vi "Add VI.vi"(8 "error in (no error)":errorcluster, 10 "Path":path, 11 "Project in":refnum<class "Project.lvclass">) -> (0 "error out":errorcluster, 3 "Project out":refnum<class "Project.lvclass">)   [LabVIEW 2015, in "Project.lvclass"]
uses:
  Project.lvclass
  Project.lvclass/Project.ctl
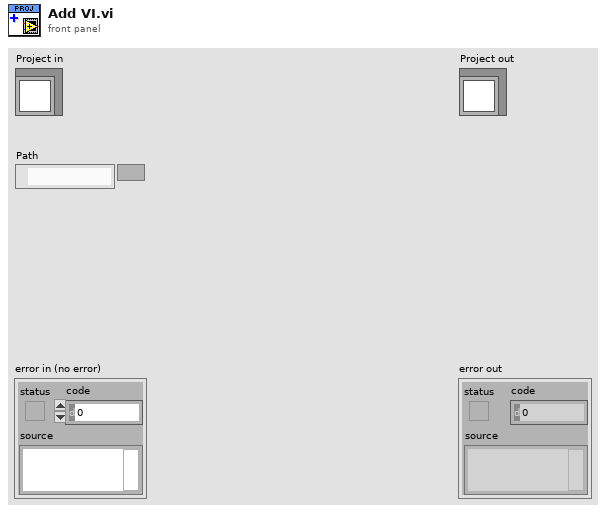
[diagram p1: front panel]
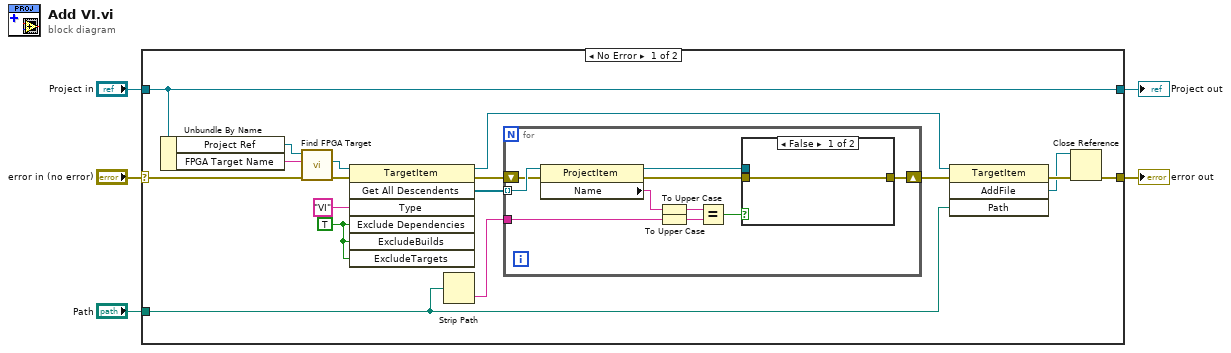
[diagram p0: block diagram]
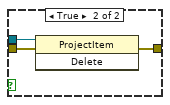
[diagram p2: hidden frame]
diagram:
  n1 = case shown="No Error" "error in (no error)" {
    selector: "error in (no error)" -> [w19 w38]
    tunnel: [w17 w38] -> w4
    tunnel: [w22 w37] -> w2
    tunnel: "Project in" -> [w22 w37]
    tunnel: "Path" -> [w8 _]
    frame No Error {
      w13 = TRUE ("ExcludeDependencies")
      n2 = Unbundle By Name(w22) -> ("Project Ref"=w21:refnum<vi>, "FPGA Target Name"=w20:string)
      n3 = call "Find FPGA Target.vi"("error in (no error)"=w19, "FPGA Target Name"=w20, "Project in"=w21) -> ("error out"=w15:errorcluster, "TargetItem out"=w11:refnum<vi>)  [unwired: 6 in, 1 out]
      n4 = invoke class="TargetItem" method="Get All Descendents"(reference=w11, error in=w15, "Type"="VI", "Exclude Dependencies"=w13, "ExcludeBuilds"=w13, "ExcludeTargets"=w13) -> (reference out=w10:refnum<vi>, error out=w9:errorcluster, "All Descendents"=w12:refnum<vi>[])  [unwired: 1 in, 4 out]
      n5 = Strip Path(path=w8) -> (name=w7:string)  [unwired: 1 out]
      n6 = for {
        tunnel: w12 -> [w32] mode=indexing
        shift-right: [w24] -> w6
        shift-left: w9 -> [w31]
        tunnel: w7 -> [w29]
        n7 = property class="ProjectItem"(reference=w32, error in=w31) -> (reference out=w26:refnum<vi>, error out=w25:errorcluster, "Name"=w30:string)
        n8 = To Upper Case(1:w30) -> (0:w28:string)
        n9 = To Upper Case(1:w29) -> (0:w27:string)
        n10 = Equal?(x=w28, y=w27) -> (x = y?=w23:bool)
        n11 = case shown="False" w23 {
          tunnel: w26 -> [_ w36]
          tunnel: w25 -> [w33 w35]
          tunnel: [w33 w34] -> w24
          frame False {
          }
          frame True {
            n12 = invoke class="ProjectItem" method="Delete"(reference=w36, error in=w35) -> (error out=w34:errorcluster)  [unwired: 1 in, 2 out]
          }
        }
      }
      n13 = invoke class="TargetItem" method="AddFile"(reference=w10, error in=w6, "Path"=w8) -> (error out=w18:errorcluster, "AddFile"=w16:refnum<vi>)  [unwired: 1 in, 2 out]
      n14 = Close Reference(reference=w16, error in (no error)=w18) -> (error out=w17:errorcluster)
    }
    frame Error {
    }
  }
  "error out" <- w4
  "Project out" <- w2
